vi "SlowCtrl.vi"(8 "Oscilloscope Ref":refnum<vi>, 9 "queue in":T1, 10 "notifier in":T2) -> ()   [LabVIEW 2012]
uses:
  TypeDefs/QueueNotifier/Notifier.ctl
  TypeDefs/QueueNotifier/DataQueue.ctl
  TypeDefs/DataTypes/SystemStatus.ctl
  TypeDefs/DataTypes/SlowCtrlState.ctl
  TypeDefs/Paths/SlowCtrlRecentPath.ctl
  <vilib>/Platform/TimedLoop/XDataNode/nitl_modes.ctl
  TypeDefs/DataTypes/SlowCtrlData.ctl
  <vilib>/Platform/TimedLoop/XDataNode/timing_clust.ctl
  <vilib>/Platform/TimedLoop/XDataNode/wakeup.ctl
  <vilib>/Platform/TimedLoop/scheduler/LVUserAPI/_suppVIs/Create_1kHz_TSource.vi
  <vilib>/Waveform/WDTFileIO.llb/Export Waveforms To Spreadsheet File (1D).vi
  <vilib>/Platform/TimedLoop/XDataNode/XDataNode.xnode
  <vilib>/Platform/TimedLoop/XDataNode/XDNodeRunTimeDep.lvlib
panel:
  out "UNIX Time":dbl format="%_13g"
  out "Time":timestamp format="%<%H:%M:%S\n%Y/%m/%d>T"
  out "LXe":dbl
  in  "Stop":bool
  in  "File Path":path=path "D:/Xe"
  in  "Open/Close Oscilloscope":bool
  out "Heater On/Off":bool
  in  "Allow Heater On?":bool
  in  "RTD1 Setpoint":dbl=165.0
  out "Xenon Phase Diagram 2":cluster{"Y":dbl[], "Y":dbl[]}[](graph) caption="Xenon Phase Diagram"
  out "Xenon Phase Diagram 1":cluster{"Y":dbl[], "Y":dbl[]}[](graph) caption="Xenon Phase Diagram"
  out "Flow Integration":dbl(graph)
  out "LXe":dbl(slide) scale=0.0..2000.0
  out "Flow, LJ channel 4":dbl(graph)
  out "Flow Rate":dbl=-0.039480482477756595
  out "Torr 2":dbl=-0.2025818864027542
  out "Pressure 2, LJ channel 2":dbl(graph)
  out "Torr":dbl=-0.2025818864027542
  out "Pressure 1, LJ channel 8":dbl(graph)
  out "Temperature Value":dbl=-9725.85
  out "RTD 4, LJ channel 13 - Cell Top/SiPM":dbl(graph)
  out "Temperature Value 2":dbl=-9725.85
  out "RTD 3, LJ channel 12":dbl(graph)
  out "Temperature Value 4":dbl=-9725.85
  out "RTD 2, LJ channel 11":dbl(graph)
  out "Temperature":dbl=-9725.85
  out "RTD 1, LJ channel 10 - Cell Bottom":dbl(graph)
  out "Temperature Value 3":dbl=1411.5161689085326
  out "RTD 0, LJ channel 1 - Coldfinger":dbl(graph)
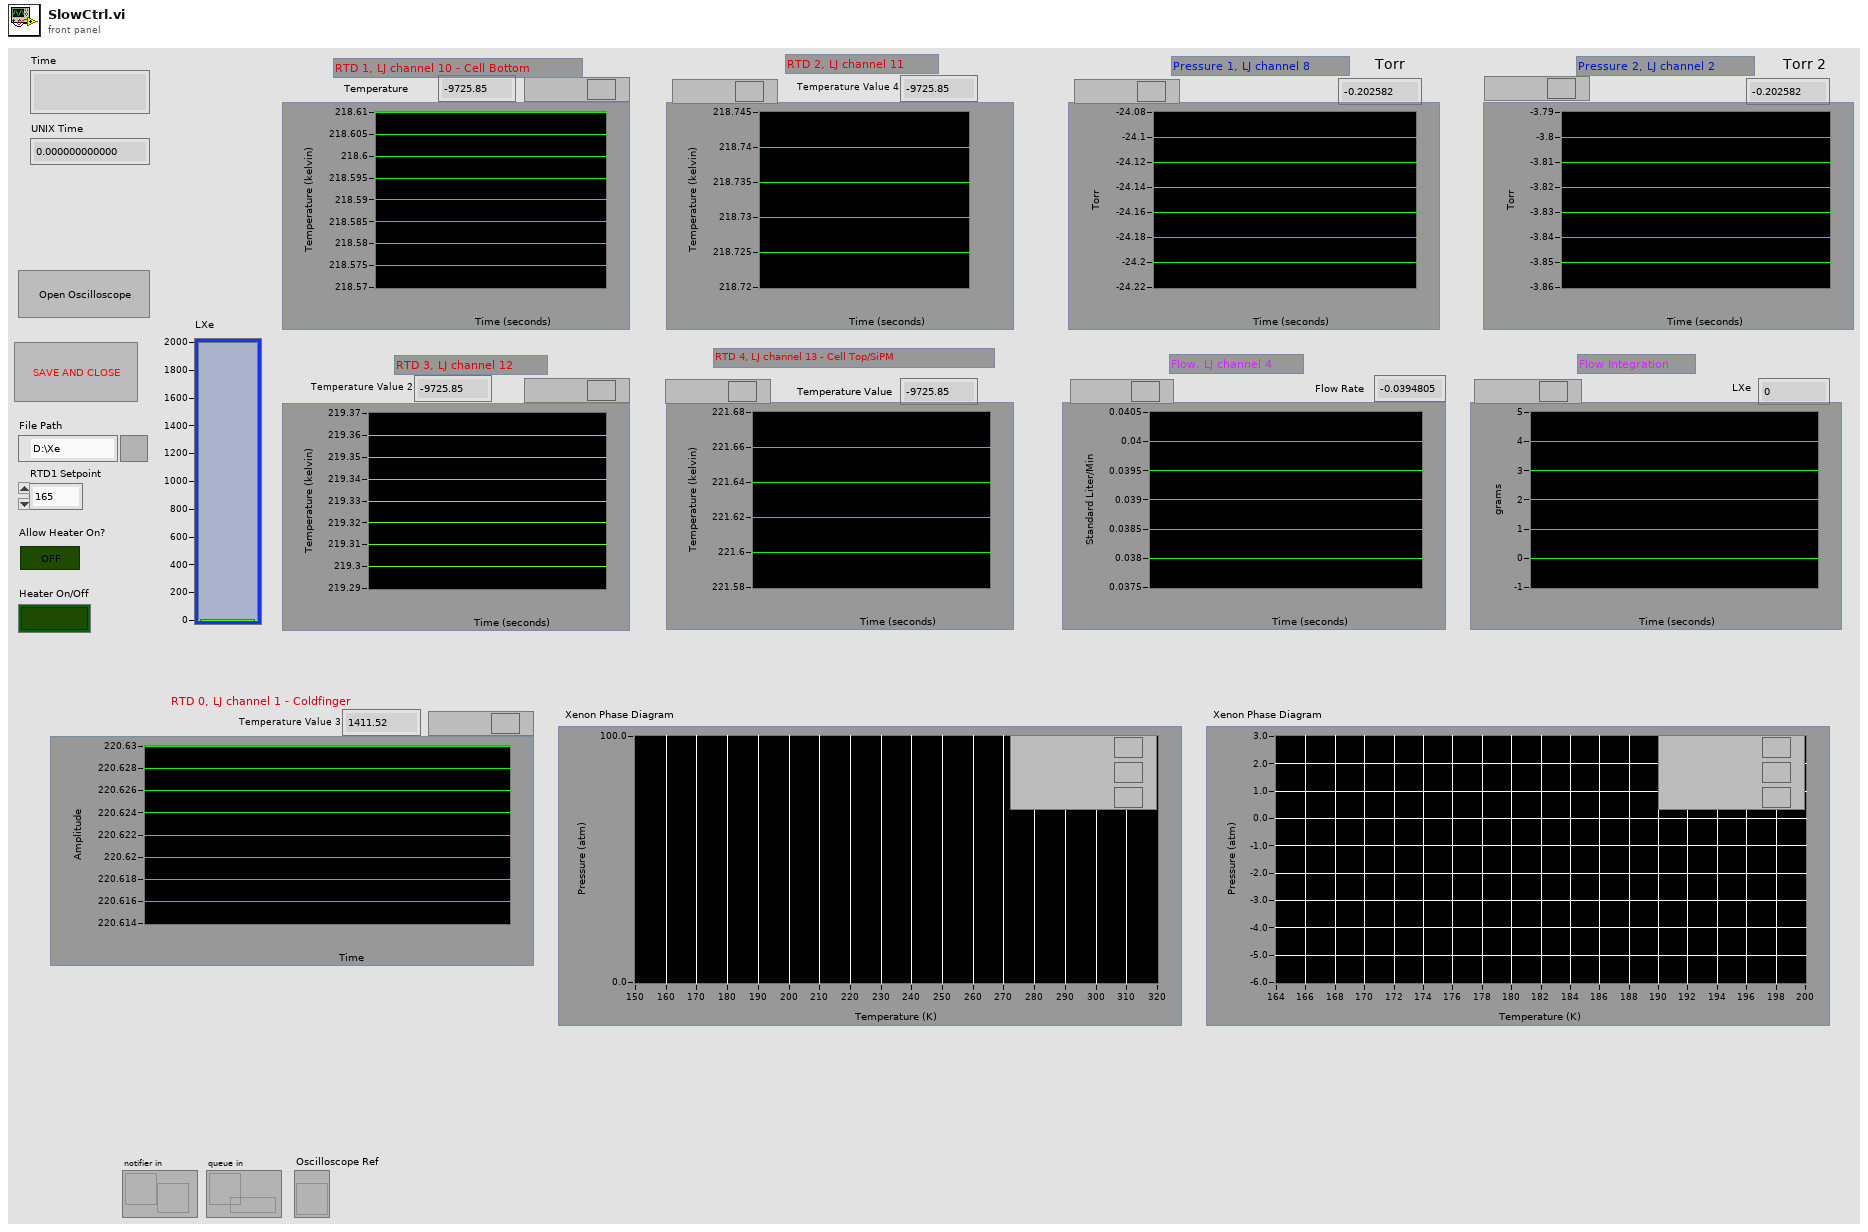
[diagram p1: front panel]
types:
  T1 = typedef "DataQueue.ctl" = refnum<queue>
  T2 = typedef "Notifier.ctl" = refnum<notifier>
  T3 = typedef "SlowCtrlRecentPath.ctl" = path
  T4 = typedef "SlowCtrlState.ctl" = enum16{"Initialize", "Run", "Shutdown"}
  T5 = typedef "SlowCtrlData.ctl" = cluster{"RTD 0":dbl, "RTD 1":dbl, "RTD 2":dbl, "RTD 3":dbl, "RTD 4":dbl, "Pressure 1":dbl, "Pressure 2":dbl, "Flow Rate":dbl, "Iteration Duration":i64}
  T6 = typedef "XDNodeRunTimeDep.lvlib/nitl_modes.ctl" = enum32{"No Change", "Process missed periods, maintain original phase", "Discard missed periods, maintain original phase", "Process missed periods, ignore original phase", "Discard missed periods, ignore original phase"}
  T7 = typedef "XDNodeRunTimeDep.lvlib/timing_clust.ctl" = cluster{"Expected End [f-1]":u64, "Actual End [f-1]":u64, "Finished Late? [f-1]":bool, "Expected End [i-1]":u64, "Actual End [i-1]":u64, "Finished Late? [i-1]":bool, "Expected Start [i]":u64, "Actual Start [i]":u64, "Expected Start [f]":u64, "Actual Start [f]":u64, "Source Name":string, "Structure Name":string, "Period":i64, "Deadline":i64, "Offset":i64, "Start":i64, "Priority":i32, "Timeout":i32, "Mode":T6, "Wakeup Reason":T8, "Error":errorcluster, "Source Type":string, "Secondary Source Type":string, "Global End Time":u64, "Global Start Time":u64, "Frame Duration":u64, "Iteration Duration":u64, "Assigned CPU":i32, "I/O Scan Engine Mode":u32}
  T8 = typedef "XDNodeRunTimeDep.lvlib/wakeup.ctl" = enum32{"Normal", "Aborted", "Asynchronous wakeup", "Timing source error", "Timed loop error", "Timeout"}
  T9 = cluster{"RTD 0, LJ channel 1 - Coldfinger":refnum<vi>, "RTD 3, LJ channel 12":refnum<vi>, "Flow Integration":refnum<vi>, "RTD 1, LJ channel 10 - Cell Bottom":refnum<vi>, "Pressure 1, LJ channel 8":refnum<vi>, "RTD 2, LJ channel 11":refnum<vi>, "RTD 4, LJ channel 13 - Cell Top/SiPM":refnum<vi>, "Flow, LJ channel 4":refnum<vi>, "Pressure 2, LJ channel 2":refnum<vi>}
  T10 = typedef "LabJackConfig.ctl" = cluster{"Negative Channels 2":i32[], "Positive Channels 2":i32[], "Handle Out":i32, "error out":errorcluster, "IO Types Out":i32[]}
  T11 = typedef "SystemStatus.ctl" = cluster{"Bias Voltage":dbl, "SiPM Temperature":dbl[], "Slow Control User":string, "LXe":dbl}
  T12 = cluster{"seconds since 1Jan1904":timestamp, "History Data":dbl[][], "LXe":dbl}
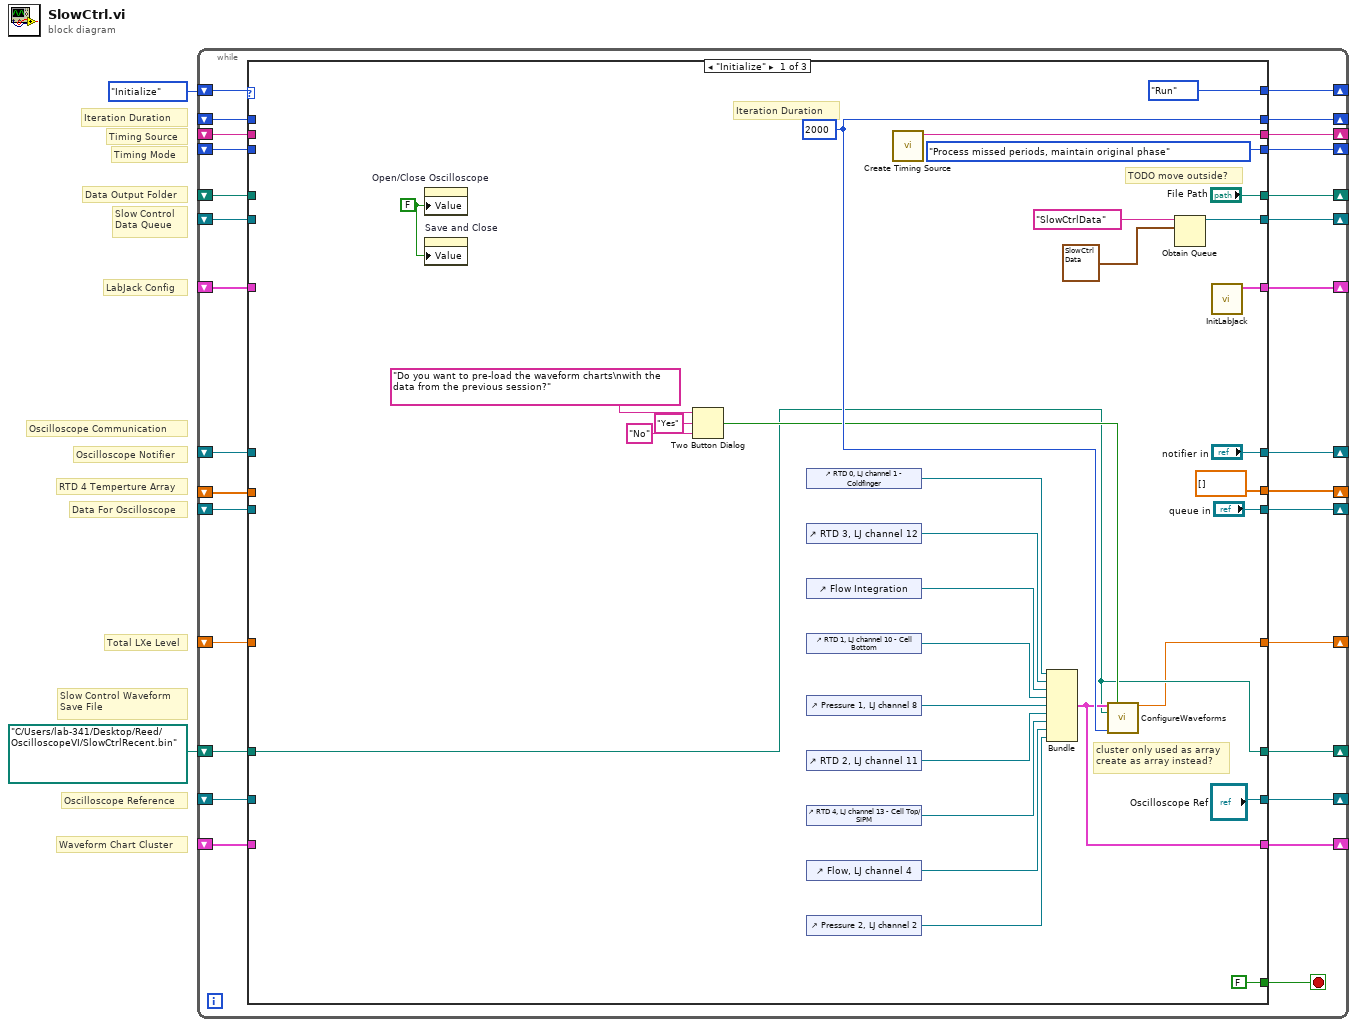
[diagram p0: block diagram]
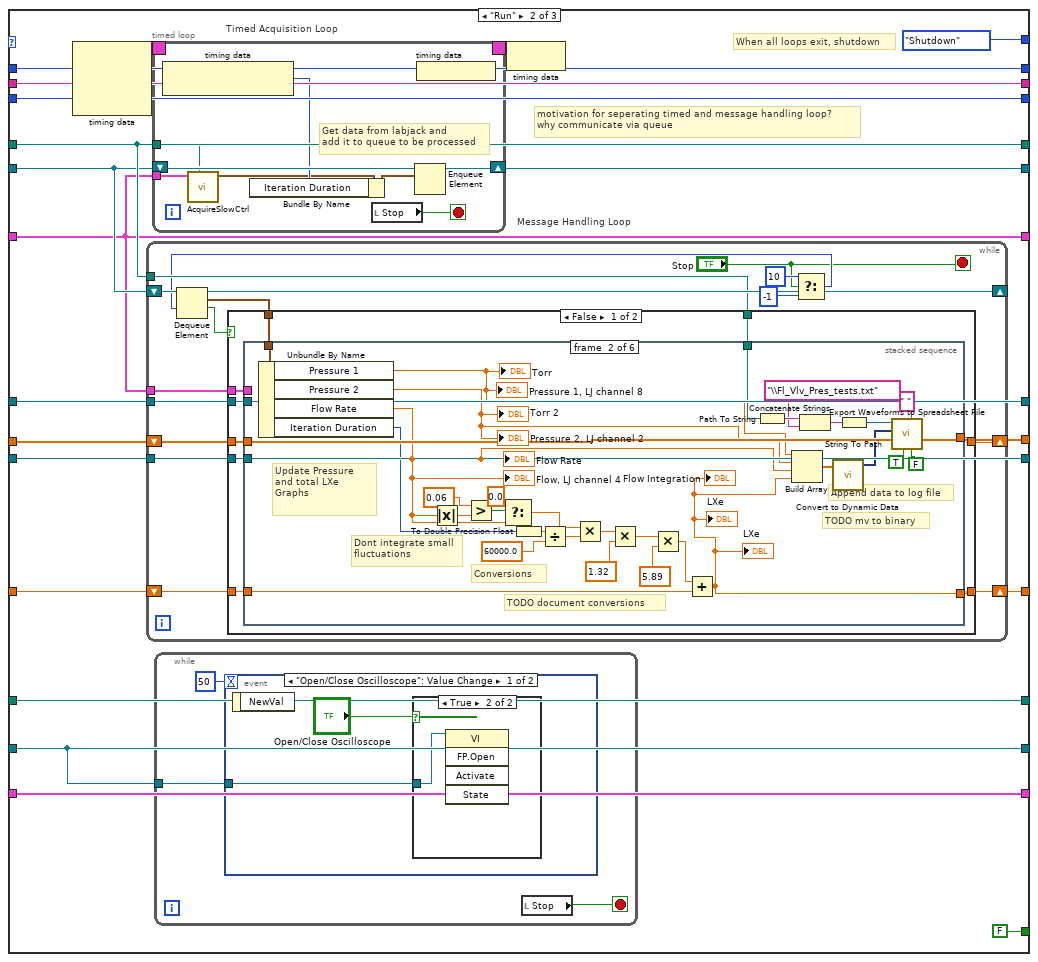
[diagram p2: hidden frame]
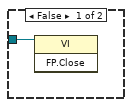
[diagram p3: hidden frame]
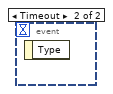
[diagram p4: hidden frame]
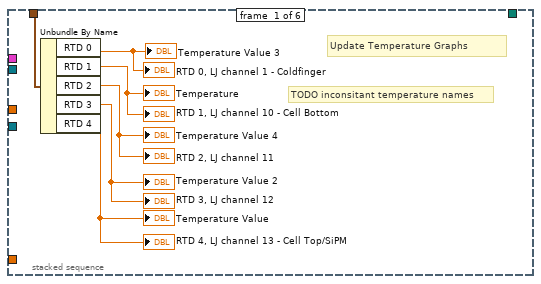
[diagram p5: hidden frame]
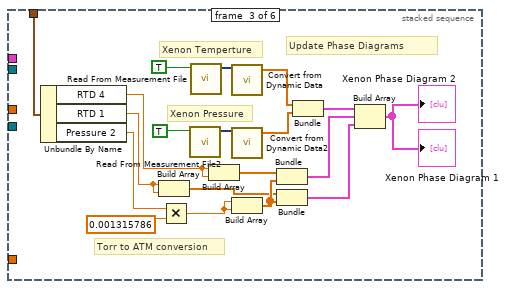
[diagram p6: hidden frame]
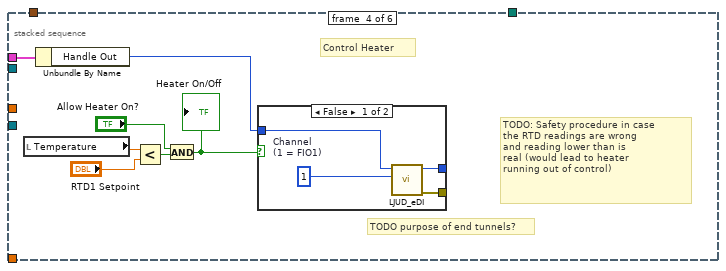
[diagram p7: hidden frame]
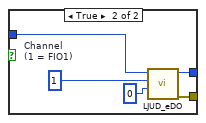
[diagram p8: hidden frame]
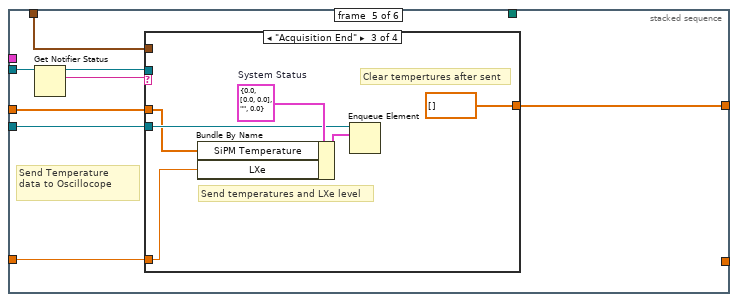
[diagram p9: hidden frame]
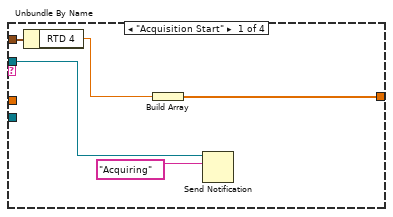
[diagram p10: hidden frame]
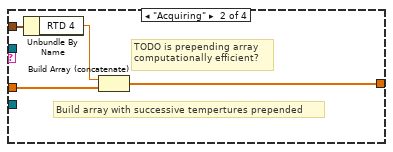
[diagram p11: hidden frame]
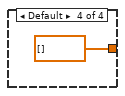
[diagram p12: hidden frame]
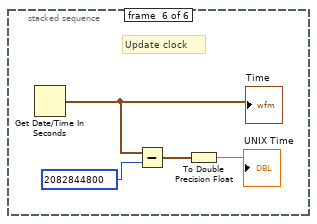
[diagram p13: hidden frame]
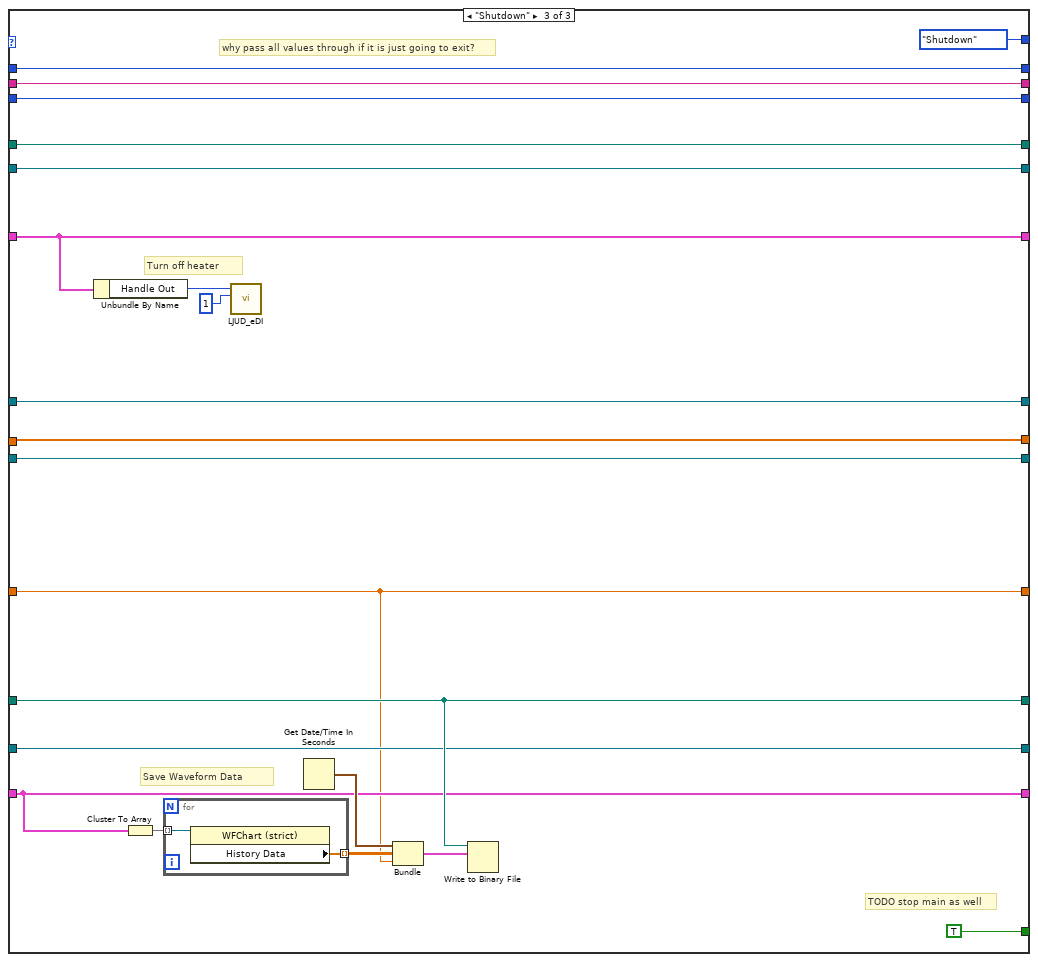
[diagram p15: hidden frame]
diagram:
  # "Oscilloscope Communication"
  # "RTD 4 Temperture Array"
  # "Data For Oscilloscope"
  # "Oscilloscope Notifier"
  # "Oscilloscope Reference"
  # "LabJack Config"
  # "Slow Control \nData Queue"
  # "Slow Control Waveform\nSave File"
  # "Timing Mode"
  # "Waveform Chart Cluster"
  # "Data Output Folder"
  # "Timing Source"
  # "Total LXe Level"
  # "Iteration Duration"
  n1 = while {
    shift-right: [w21] -> _
    shift-left: _ -> [w24]
    shift-right: [w22] -> _
    shift-left: _ -> [w31]
    shift-right: [w19] -> _
    shift-left: _ -> [w30]
    shift-right: [w20] -> _
    shift-left: _ -> [w23]
    shift-right: [w14] -> _
    shift-left: _ -> [w25]
    shift-right: [w13] -> _
    shift-left: _ -> [w27]
    shift-right: [w12] -> _
    shift-left: _ -> [w26]
    shift-right: [w11] -> _
    shift-left: _ -> [w29]
    shift-right: [w10] -> _
    shift-left: _ -> [w28]
    shift-right: [w18] -> _
    shift-left: _ -> [w17]
    shift-right: [w16] -> _
    shift-left: _ -> [w15]
    shift-right: [w9] -> _
    shift-left: SlowCtrlState."Initialize" -> [w8]
    shift-right: [w7] -> _
    shift-left: _ -> [w6]
    shift-right: [w4] -> _
    shift-left: T3 path "C:/Users/lab-341/Desktop/Reed/OscilloscopeVI/SlowCtrlRecent.bin" ("path") -> [w5]
    stop <- w3 stop-if-true
    n2 = case shown="\"Initialize\"" w8 {
      tunnel: w31 -> [_ w75 w240]
      tunnel: w30 -> [_ w74 w241]
      tunnel: w29 -> [_ w67 w231]
      tunnel: w28 -> [_ w65 w236]
      tunnel: w27 -> [_ w69 w245]
      tunnel: w26 -> [_ w68 w246]
      tunnel: w25 -> [_ w70 w244]
      tunnel: w24 -> [_ w76 w239]
      tunnel: w23 -> [_ w73 w242]
      tunnel: [w51 w75 w240] -> w22
      tunnel: [w38 w76 w239] -> w21
      tunnel: ["File Path" w73 w242] -> w20
      tunnel: [nitl_modes."Process missed periods, maintain original phase" ("Mode") w74 w241] -> w19
      tunnel: [w48 w71 w234] -> w18
      tunnel: w17 -> [_ w71 w234]
      tunnel: [w47 w72 w243] -> w16
      tunnel: w15 -> [_ w72 w243]
      tunnel: ["notifier in" w70 w244] -> w14
      tunnel: ["queue in" w69 w245] -> w13
      tunnel: [dbl[] [] w68 w246] -> w12
      tunnel: [w32 w63 w231] -> w11
      tunnel: ["Oscilloscope Ref" w65 w236] -> w10
      tunnel: [SlowCtrlState."Run" SlowCtrlState."Shutdown" SlowCtrlState."Shutdown"] -> w9
      tunnel: [w37 w64 w235] -> w7
      tunnel: w6 -> [_ w64 w235]
      tunnel: w5 -> [w33 w66 w237]
      tunnel: [w33 w66 w237] -> w4
      tunnel: [FALSE FALSE TRUE] -> w3
      frame "Initialize" {
        w36 = FALSE ("Open/Close Oscilloscope")
        w38 = i64 2000 ("Period")
        # "TODO move outside?"
        # "cluster only used as array\ncreate as array instead?"
        # "Iteration Duration"
        n3 = property on="Open/Close Oscilloscope" class="Bool (strict)"("Value"=w36) -> ()  [unwired: 2 in, 2 out]
        n4 = property on="Save and Close" class="Bool (strict)"("Value"=w36) -> ()  [unwired: 2 in, 2 out]
        n5 = Two Button Dialog(message="Do you want to pre-load the waveform charts\nwith the data from the previous session?", 1:"No" ("F button name (\"Cancel\")"), 2:"Yes" ("T button name (\"OK\")")) -> (T button?=w34:bool)
        n6 = control-ref of="RTD 0, LJ channel 1 - Coldfinger"() -> (w54:refnum<vi>)
        n7 = control-ref of="RTD 3, LJ channel 12"() -> (w55:refnum<vi>)
        n8 = control-ref of="Flow Integration"() -> (w56:refnum<vi>)
        n9 = control-ref of="RTD 1, LJ channel 10 - Cell Bottom"() -> (w57:refnum<vi>)
        n10 = control-ref of="Pressure 1, LJ channel 8"() -> (w58:refnum<vi>)
        n11 = control-ref of="RTD 2, LJ channel 11"() -> (w59:refnum<vi>)
        n12 = control-ref of="RTD 4, LJ channel 13 - Cell Top/SiPM"() -> (w60:refnum<vi>)
        n13 = control-ref of="Flow, LJ channel 4"() -> (w61:refnum<vi>)
        n14 = control-ref of="Pressure 2, LJ channel 2"() -> (w62:refnum<vi>)
        n15 = call-poly <vilib>:"Create Timing Source.vi"() -> ("name (out)"=w51:string)  [unwired: 10 in, 1 out]
        n16 = Bundle("RTD 0, LJ channel 1 - Coldfinger"=w54, "RTD 3, LJ channel 12"=w55, "Flow Integration"=w56, "RTD 1, LJ channel 10 - Cell Bottom"=w57, "Pressure 1, LJ channel 8"=w58, "RTD 2, LJ channel 11"=w59, "RTD 4, LJ channel 13 - Cell Top/SiPM"=w60, "Flow, LJ channel 4"=w61, "Pressure 2, LJ channel 2"=w62) -> (w37:T9)  [unwired: 1 in]
        n17 = call "ConfigureWaveforms.vi"("WFReferences"=w37, "PreLoad Charts?"=w34, "path"=w33, "Iteration Duration"=w38) -> ("LXe"=w32:dbl)  [unwired: 11 in]
        n18 = Obtain Queue(name (unnamed)="SlowCtrlData", element data type=T5 {"RTD 0"=0.0, "RTD 1"=0.0, "RTD 2"=0.0, "RTD 3"=0.0, "RTD 4"=0.0, "Pressure 1"=0.0, "Pressure 2"=0.0, "Flow Rate"=0.0, "Iteration Duration"=0} ("Slow Control Data")) -> (queue out=w47:refnum<queue>)  [unwired: 3 in, 2 out]
        n19 = call "InitLabJack.vi"() -> ("LJConfig"=w48:T10)  [unwired: 11 in]
      }
      frame "Run" {
        # "motivation for seperating timed and message handling loop?\nwhy communicate via queue"
        # "When all loops exit, shutdown"
        n20 = node-c288(w76, w75, w74) -> (w80:T7)
        n21 = while "Message Handling Loop" {
          shift-right: [w103] -> _
          shift-left: w72 -> [w102]
          shift-right: [w101] -> w63
          shift-left: w67 -> [w100]
          tunnel: w71 -> [w99]
          tunnel: w69 -> [w95]
          shift-right: [w98] -> _
          shift-left: w68 -> [w97]
          tunnel: w70 -> [w96]
          tunnel: w73 -> [w94]
          stop <- "Stop" stop-if-true
          n22 = Select(t=10 ("timeout in ms (-1)"), s="Stop", f=-1 ("timeout in ms (-1)")) -> (s? t:f=w92:i32)
          n23 = Dequeue Element(queue=w102, timeout in ms (-1)=w92) -> (queue out=w103:refnum<queue>, element=w89:T5, timed out?=w90:bool)  [unwired: 1 in, 1 out]
          n24 = case shown="False" w90 {
            tunnel: [w112 w212] -> w101
            tunnel: w100 -> [w111 w212]
            tunnel: w99 -> [w110 _]
            tunnel: [w109 w213] -> w98
            tunnel: w97 -> [w108 w213]
            tunnel: w96 -> [w107 _]
            tunnel: w95 -> [w106 _]
            tunnel: w94 -> [w105 _]
            tunnel: w89 -> [w104 _]
            frame False {
              n25 = stacked-sequence {
                tunnel: w104 -> [w113 w148 w167 _ w189 _]
                tunnel: [_ w123 _ _ _ _] -> w112
                tunnel: w111 -> [_ w134 _ _ w184 _]
                tunnel: w110 -> [_ _ _ w174 _ _]
                tunnel: w107 -> [_ _ _ _ w190 _]
                tunnel: w108 -> [_ _ _ _ w188 _]
                tunnel: [_ _ _ _ w187 _] -> w109
                tunnel: w106 -> [_ _ _ _ w186 _]
                tunnel: w105 -> [_ w124 _ _ _ _]
                frame #0 {
                  # "TODO inconsitant temperature names"
                  # "Update Temperature Graphs"
                  n26 = Unbundle By Name(w113) -> ("RTD 0"=→"RTD 0, LJ channel 1 - Coldfinger" →"Temperature Value 3":dbl, "RTD 1"=→"RTD 1, LJ channel 10 - Cell Bottom" →"Temperature":dbl, "RTD 2"=→"RTD 2, LJ channel 11" →"Temperature Value 4":dbl, "RTD 3"=→"RTD 3, LJ channel 12" →"Temperature Value 2":dbl, "RTD 4"=→"RTD 4, LJ channel 13 - Cell Top/SiPM" →"Temperature Value":dbl)
                }
                frame #1 {
                  # "TODO mv to binary"
                  # "TODO document conversions"
                  # "Append data to log file"
                  # "Dont integrate small\nfluctuations"
                  # "Update Pressure\nand total LXe \nGraphs"
                  # "Conversions"
                  n27 = Unbundle By Name(w148) -> ("Pressure 1"=w122:dbl, "Pressure 2"=w121:dbl, "Flow Rate"=w119:dbl, "Iteration Duration"=w140:i64)
                  "Pressure 1, LJ channel 8" <- w122
                  "Torr" <- w122
                  "Pressure 2, LJ channel 2" <- w121
                  "Torr 2" <- w121
                  "Flow Rate" <- w119
                  "Flow, LJ channel 4" <- w119
                  n28 = Absolute Value(x=w119) -> (abs(x)=w120:dbl)
                  n29 = Greater?(x=0.06 ("y"), y=w120) -> (0:w138:bool)
                  n30 = Select(t=0.0, s=w138, f=w119) -> (s? t:f=w137:dbl)
                  n31 = To Double Precision Float(number=w140) -> (double precision float=w142:dbl)
                  n32 = Divide(x=w142, y=60000.0) -> (x/y=w143:dbl)
                  n33 = Multiply(x=w137, y=w143) -> (x*y=w144:dbl)
                  n34 = Multiply(x=w144, y=1.32) -> (x*y=w145:dbl)
                  n35 = Multiply(x=w145, y=5.89) -> (x*y=w135:dbl)
                  n36 = Add(x=w135, y=w134) -> (x+y=w123:dbl)
                  "LXe" <- w123
                  "Flow Integration" <- w123
                  "LXe" <- w123
                  n37 = Path To String(path=w124) -> (string=w131:string)
                  n38 = Build Array(w122, w121, w119, w123) -> (w130:dbl[])
                  n39 = Concatenate Strings(w131, "\\Fl_Vlv_Pres_tests.txt") -> (w127:string)
                  n40 = call "Convert to Dynamic Data"("Array"=w130) -> ("Dynamic Data Type"=w125:dynamicdata)  [unwired: 3 in]
                  n41 = String To Path(string=w127) -> (path=w128:path)
                  n42 = call-poly <vilib>:"Export Waveforms to Spreadsheet File.vi"("header? (write header:T)"=FALSE, "delimiter (Tab)"=" ", "append to file? (new file:F)"=TRUE, "waveforms"=w125, "file path (dialog if empty)"=w128) -> ()  [unwired: 5 in, 2 out]
                }
                frame #2 {
                  # "Xenon Pressure"
                  # "Xenon Temperture"
                  # "Torr to ATM conversion"
                  # "Update Phase Diagrams"
                  n43 = Unbundle By Name(w167) -> ("RTD 4"=w152:dbl, "RTD 1"=w151:dbl, "Pressure 2"=w150:dbl)
                  n44 = Build Array(w151, w151) -> (w155:dbl[])
                  n45 = Multiply(x=w150, y=0.001315786) -> (x*y=w149:dbl)
                  n46 = call "Read From Measurement File2"("Reset"=TRUE) -> ("Signals"=w164:dynamicdata)  [unwired: 5 in, 5 out]
                  n47 = call "Read From Measurement File"("Reset"=TRUE) -> ("Signals"=w163:dynamicdata)  [unwired: 5 in, 5 out]
                  n48 = Build Array(w152, w152) -> (w156:dbl[])
                  n49 = call "Convert from Dynamic Data"("Dynamic Data Type"=w163) -> ("Array"=w162:dbl[])  [unwired: 3 in]
                  n50 = call "Convert from Dynamic Data2"("Dynamic Data Type"=w164) -> ("Array"=w161:dbl[])  [unwired: 3 in]
                  n51 = Build Array(w149, w149) -> (w157:dbl[])
                  n52 = Bundle(w156, w157) -> (w159:cluster{dbl[], dbl[]})  [unwired: 1 in]
                  n53 = Bundle(w155, w157) -> (w158:cluster{dbl[], dbl[]})  [unwired: 1 in]
                  n54 = Bundle("Array"=w162, "Array"=w161) -> (w160:cluster{"Array":dbl[], "Array":dbl[]})  [unwired: 1 in]
                  n55 = Build Array(w160, w159, w158) -> (→"Xenon Phase Diagram 1" →"Xenon Phase Diagram 2":cluster{"Array":dbl[], "Array":dbl[]}[])
                }
                frame #3 {
                  # "TODO purpose of end tunnels?"
                  # "TODO: Safety procedure in case\nthe RTD readings are wrong\nand reading lower than is\nreal (would lead to heater\nrunning out of control)"
                  # "Control Heater"
                  n56 = local read "Temperature"() -> (w169:dbl)
                  n57 = Unbundle By Name(w174) -> ("Handle Out"=w168:i32)
                  n58 = Less?(x=w169, y="RTD1 Setpoint") -> (x < y?=w171:bool)
                  n59 = And(x="Allow Heater On?", y=w171) -> (x .and. y?=w173:bool)
                  "Heater On/Off" <- w173
                  n60 = case shown="False" w173 {
                    tunnel: [w177 w181] -> _
                    tunnel: [w176 w180] -> _
                    tunnel: w168 -> [w175 w179]
                    frame False {
                      w178 = 1  # Channel (1 = FIO1)
                      n61 = call <vilib>:"LJUD_eDI.vi"("Channel"=w178, "Handle In"=w175) -> ("error out"=w177:errorcluster, "Handle Out"=w176:i32)  [unwired: 7 in, 1 out]
                    }
                    frame True {
                      w182 = 1  # Channel (1 = FIO1)
                      n62 = call <vilib>:"LJUD_eDO.vi"("State"=0, "Channel"=w182, "Handle In"=w179) -> ("error out"=w181:errorcluster, "Handle Out"=w180:i32)  [unwired: 7 in]
                    }
                  }
                }
                frame #4 {
                  # "Send Temperature\ndata to Oscillocope"
                  n63 = Get Notifier Status(notifier=w190) -> (notifier out=w191:T2, current notification=w185:string)  [unwired: 1 in, 3 out]
                  n64 = case shown="\"Acquisition End\"" w185 {
                    tunnel: [w196 w200 dbl[] [] dbl[] []] -> w187
                    tunnel: w191 -> [w195 _ _ _]
                    tunnel: w189 -> [w193 w199 _ _]
                    tunnel: w188 -> [_ w197 w202 _]
                    tunnel: w186 -> [_ _ w203 _]
                    tunnel: w184 -> [_ _ w201 _]
                    frame "Acquisition Start" {
                      n65 = Unbundle By Name(w193) -> ("RTD 4"=w192:dbl)
                      n66 = Build Array(w192) -> (w196:dbl[])
                      n67 = Send Notification(notification="Acquiring", notifier=w195) -> ()  [unwired: 1 in, 2 out]
                    }
                    frame "Acquiring" {
                      # "TODO is prepending array\ncomputationally efficient?"
                      # "Build array with successive tempertures prepended"
                      n68 = Unbundle By Name(w199) -> ("RTD 4"=w198:dbl)
                      n69 = Build Array (concatenate)(w198, w197) -> (w200:dbl[])
                    }
                    frame "Acquisition End" {
                      w205 = T11 {"Bias Voltage"=0.0, "SiPM Temperature"=[0.0, 0.0], "Slow Control User"="", "LXe"=0.0}  # System Status
                      # "Send temperatures and LXe level"
                      # "Clear tempertures after sent"
                      n70 = Bundle By Name(cluster=w205, "SiPM Temperature"=w202, "LXe"=w201) -> (w204:T11)
                      n71 = Enqueue Element(queue=w203, element=w204) -> ()  [unwired: 2 in, 3 out]
                    }
                    frame Default {
                    }
                  }
                }
                frame #5 {
                  # "Update clock"
                  n72 = Get Date/Time In Seconds() -> (seconds since 1Jan1904=w208:timestamp)
                  "Time" <- w208
                  n73 = Subtract(x=w208, y=2082844800) -> (x-y=w210:timestamp)
                  n74 = To Double Precision Float(number=w210) -> (double precision float=→"UNIX Time":dbl)
                }
              }
            }
            frame True {
              # "Wait for new data to be collected and added to queue"
            }
          }
        }
        n75 = timed-loop "Timed Acquisition Loop" {
          tunnel: w71 -> [w221]
          shift-right: [w220] -> _
          shift-left: w72 -> [w219]
          timing: w80 -> [_]
          timing-out: [_] -> w79
          tunnel: w73 -> [w217]
          stop <- w216 stop-if-true
          # "Get data from labjack and\nadd it to queue to be processed"
          n76 = node-c288() -> (w215:i64)  [unwired: 1 in]
          n77 = call "AcquireSlowCtrl.vi"("File Path"=w217, "LJConfig In"=w221) -> ("Slow Control Data"=w214:T5)  [unwired: 9 in]
          n78 = Bundle By Name(cluster=w214, "Iteration Duration"=w215) -> (w218:T5)
          n79 = local read "Stop"() -> (w216:bool)
          n80 = Enqueue Element(queue=w219, element=w218) -> (queue out=w220:refnum<queue>)  [unwired: 2 in, 2 out]
          n81 = node-c288() -> ()  [unwired: 1 out]
        }
        n82 = while {
          tunnel: w65 -> [w83]
          stop <- w82 stop-if-true
          n83 = event shown="[0] \"Open/Close Oscilloscope\": Value Change" {
            selector: _ -> [_ _]
            dyn-events: _ -> [_ _]
            timeout: 50 -> [_ _]
            tunnel: w83 -> [w84 _]
            event "Open/Close Oscilloscope": Value Change {
              n84 = event-data() -> ()  [unwired: 1 in, 1 out]
              n85 = case shown="True" "Open/Close Oscilloscope" {
                tunnel: w84 -> [w86 w87]
                frame False {
                  n86 = invoke class="VI" method="FP.Close"(reference=w86) -> ()  [unwired: 2 in, 3 out]
                }
                frame True {
                  n87 = invoke class="VI" method="FP.Open"(reference=w87) -> ()  [unwired: 4 in, 5 out]
                }
              }
            }
            event Timeout {
              n88 = event-data() -> ()  [unwired: 1 in, 1 out]
            }
          }
          n89 = local read "Stop"() -> (w82:bool)
        }
        n90 = node-c288(w79) -> ()
      }
      frame "Shutdown" {
        # "Turn off heater"
        # "TODO stop main as well"
        # "why pass all values through if it is just going to exit?"
        # "Save Waveform Data"
        n91 = Unbundle By Name(w234) -> ("Handle Out"=w233:i32)
        n92 = Cluster To Array(cluster=w235) -> (array=w251:refnum<vi>[])
        n93 = for {
          tunnel: w251 -> [w253] mode=indexing
          tunnel: [w252] -> w249 mode=indexing
          n94 = property on="Property Node" class="WFChart (strict)"(reference=w253) -> ("History Data"=w252:dbl[])  [unwired: 1 in, 2 out]
        }
        n95 = call <vilib>:"LJUD_eDI.vi"("Channel"=1, "Handle In"=w233) -> ()  [unwired: 7 in, 3 out]
        n96 = Get Date/Time In Seconds() -> (seconds since 1Jan1904=w250:timestamp)
        n97 = Bundle("seconds since 1Jan1904"=w250, "History Data"=w249, "LXe"=w231) -> (w248:T12)  [unwired: 1 in]
        n98 = Write to Binary File(file (use dialog)=w237, data=w248) -> ()  [unwired: 4 in, 3 out]
      }
    }
  }
